vi "OscTest.vi"() -> ()   [LabVIEW 2017]
uses:
  <vilib>/Analysis/baseanly.llb/Mean (DBL).vi
  DS1054z.lvlib
  <vilib>/Analysis/NI_AALBase.lvlib
panel:
  out "Waveform Chart":u32(graph)
  out "Array":string[](array[string])
  out "OutData":cluster{string, "userdata":string}
  out "Waveform Graph 5":dbl[](graph)
  out "Waveform Graph 4":u32[](graph)
  out "mean":dbl format="%0.2f"
  out "Waveform Graph 3":dbl[](graph)
  out "Numeric":i32
  out "x-y":u32
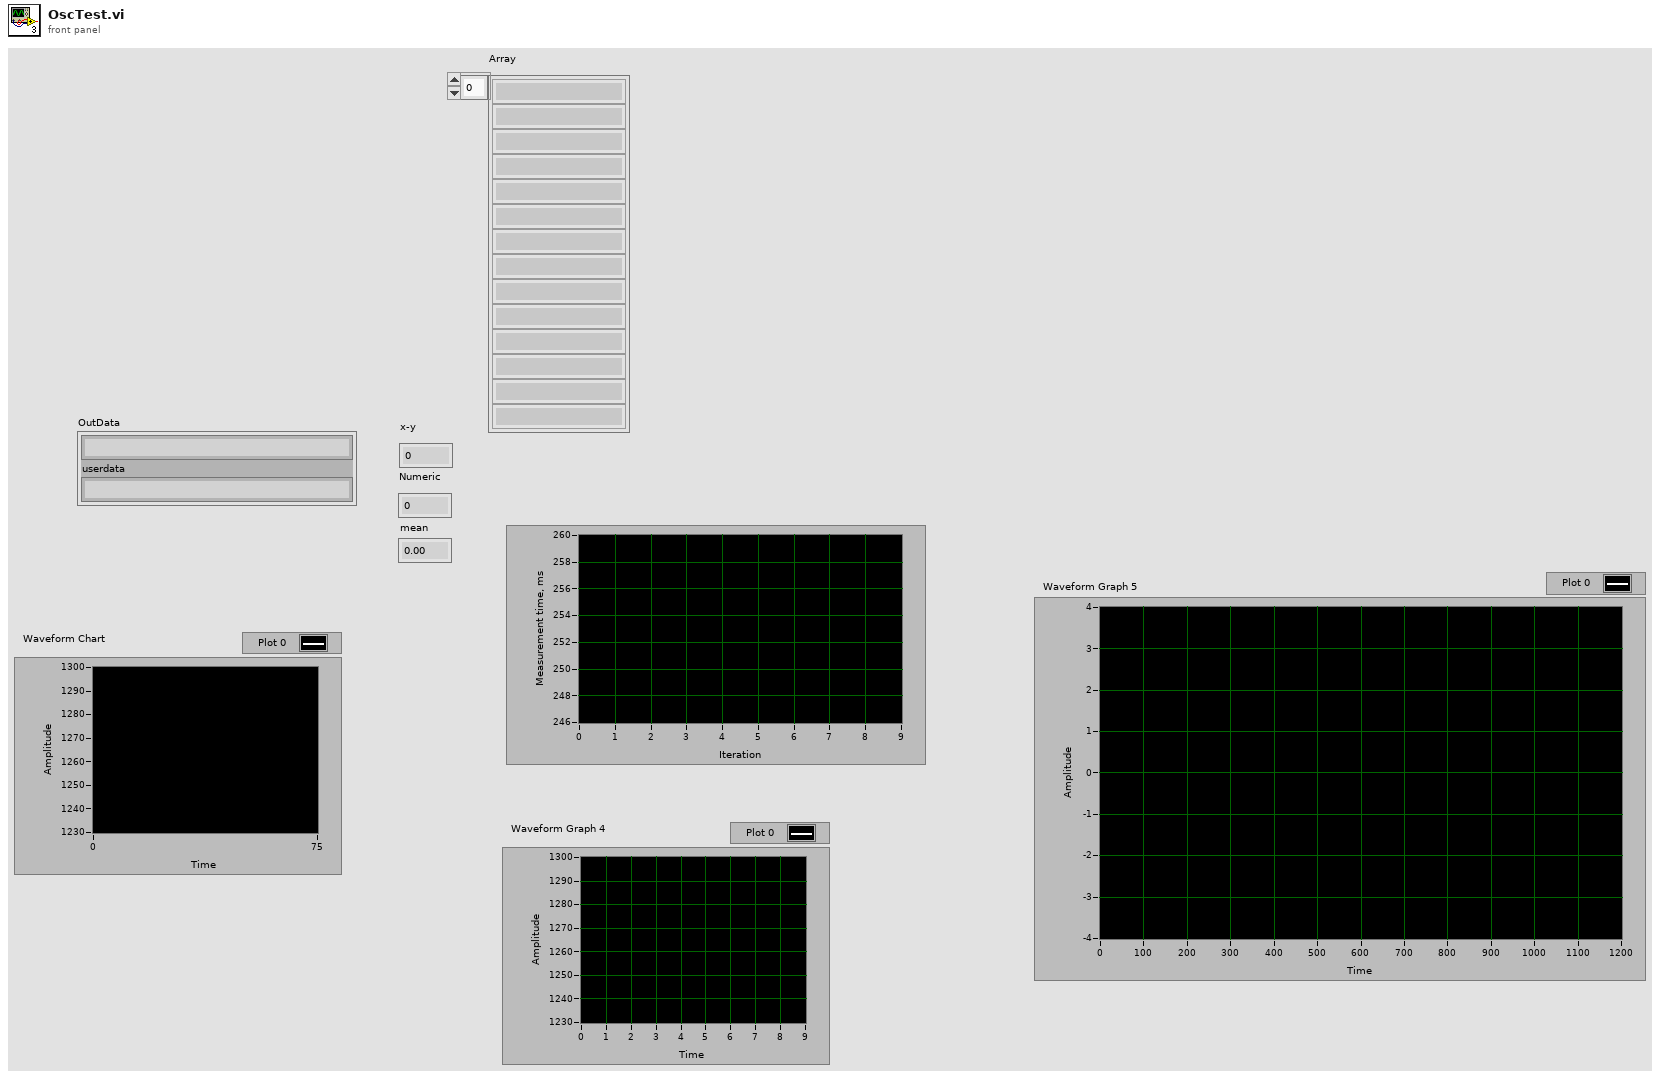
[diagram p1: front panel]
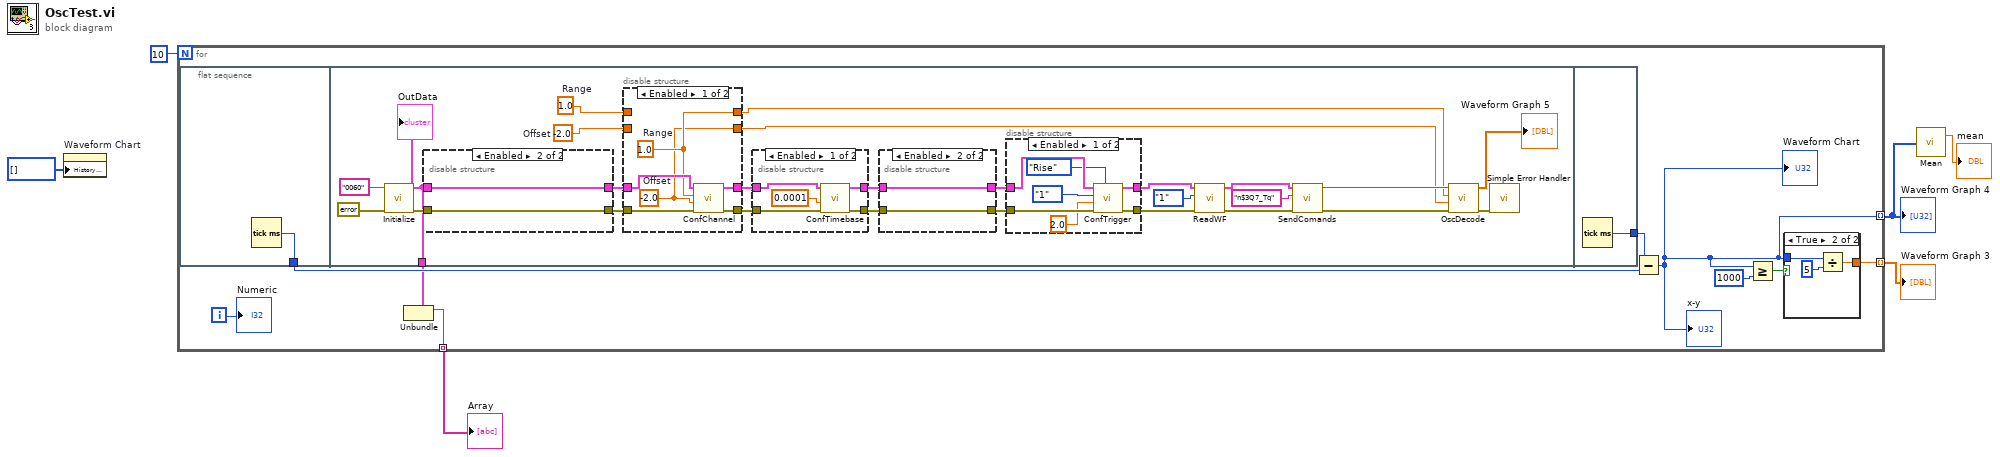
[diagram p0: block diagram]
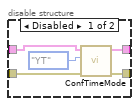
[diagram p4: hidden frame]
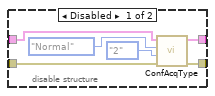
[diagram p7: hidden frame]
diagram:
  n1 = property on="Waveform Chart" class="WFChart (strict)"("History Data"=u32[] []) -> ()  [unwired: 2 in, 2 out]
  n2 = for {
    N: 10 -> [_]
    tunnel: [w7] -> w1 mode=indexing
    tunnel: [w11] -> w4 mode=indexing
    tunnel: [w9] -> w3 mode=indexing
    i -> [w14]
    n3 = flat-sequence {
      tunnel: [w20] -> w15
      tunnel: [w21] -> w10
      tunnel: [w88] -> w8
      frame #0 {
        n4 = Tick Count (ms)() -> (millisecond timer value=w20:u32)
      }
      frame #1 {
        w22 = -2.0  # Offset
        w23 = 1.0  # Range
        n5 = call "Initialize.vi"("error in (no error)"=errorcluster {"status"=FALSE, "code"=0, "source"=""}, "UserID"="0060") -> ("error out"=w44:errorcluster, "OutData"=w21:cluster{string, "userdata":string})  [unwired: 8 in]
        "OutData" <- w21
        n6 = disable-structure shown="Enabled" {
          disable-tunnel: w21 -> [w85 w87]
          disable-tunnel: w44 -> [w84 w86]
          disable-tunnel: [w81 w87] -> w37
          disable-tunnel: [w80 w86] -> w36
          frame Disabled {
            n7 = call "ConfAcqType.vi"("error in"=w84, "NumOfAver"=enum16{"2", "4", "8", "16"}."2", "Type"=enum16{"Normal", "Average", "Peak Detect"}."Normal", "InputData"=w85) -> ("error out"=w80:errorcluster, "OutputData"=w81:cluster{"String":string, string})  [unwired: 6 in]
          }
          frame Enabled {
          }
        }
        n8 = disable-structure shown="Enabled" {
          disable-tunnel: w37 -> [w75 w79]
          disable-tunnel: w36 -> [w74 w78]
          disable-tunnel: [w73 w79] -> w35
          disable-tunnel: [w72 w78] -> w34
          disable-tunnel: [w71 w77] -> w25
          disable-tunnel: [w70 w76] -> w24
          disable-tunnel: w23 -> [_ w77]
          disable-tunnel: w22 -> [_ w76]
          frame Enabled {
            w70 = -2.0  # Offset
            w71 = 1.0  # Range
            n9 = call "ConfChannel.vi"("error in"=w74, "Offset"=w70, "Range"=w71, "InputData"=w75) -> ("error out"=w72:errorcluster, "OutputData"=w73:cluster{"String":string, string})  [unwired: 6 in]
          }
          frame Disabled {
          }
        }
        n10 = disable-structure shown="Enabled" {
          disable-tunnel: w35 -> [w67 w69]
          disable-tunnel: w34 -> [w66 w68]
          disable-tunnel: [w65 w69] -> w33
          disable-tunnel: [w64 w68] -> w32
          frame Enabled {
            n11 = call "ConfTimebase.vi"("error in"=w66, "Timebase"=0.0001, "InputData"=w67) -> ("error out"=w64:errorcluster, "OutputData"=w65:cluster{"String":string, string})  [unwired: 7 in]
          }
          frame Disabled {
          }
        }
        n12 = disable-structure shown="Enabled" {
          disable-tunnel: w33 -> [w60 w62]
          disable-tunnel: w32 -> [w59 w61]
          disable-tunnel: [w58 w62] -> w31
          disable-tunnel: [w57 w61] -> w30
          frame Disabled {
            n13 = call "ConfTimeMode.vi"("error in"=w59, "Timebase Mode"=enum16{"YT", "XY"}."YT", "InputData"=w60) -> ("error out"=w57:errorcluster, "OutputData"=w58:cluster{"String":string, string})  [unwired: 7 in]
          }
          frame Enabled {
          }
        }
        n14 = disable-structure shown="Enabled" {
          disable-tunnel: [w53 w55] -> w42
          disable-tunnel: [w52 w54] -> w40
          disable-tunnel: w31 -> [w51 w55]
          disable-tunnel: w30 -> [w50 w54]
          frame Enabled {
            n15 = call "ConfTrigger.vi"("Slope"=enum16{"Rise", "Fall", "Both"}."Rise", "error in"=w50, "Level"=2.0, "Source"=enum16{"1", "2", "3", "4"}."1", "InputData"=w51) -> ("error out"=w52:errorcluster, "OutputData"=w53:cluster{"String":string, string})  [unwired: 5 in]
          }
          frame Disabled {
          }
        }
        n16 = call "ReadWF.vi"("error in"=w40, "Source"=enum16{"1", "2", "3", "4"}."1", "InputData"=w42) -> ("error out"=w39:errorcluster, "OutputData"=w41:cluster{"String":string, string})  [unwired: 7 in]
        n17 = call "SendComands.vi"("error in (no error)"=w39, "Password"="n$3Q7_Tq", "InputData"=w41) -> ("error out"=w28:errorcluster, "Result"=w29:string)  [unwired: 6 in, 1 out]
        n18 = call "OscDecode.vi"("error in"=w28, "Offset"=w24, "Range"=w25, "ReceivedData"=w29) -> ("error out"=w27:errorcluster, "MeasuredData"=→"Waveform Graph 5":dbl[])  [unwired: 5 in, 1 out]
        n19 = call <vilib>:"Simple Error Handler.vi"("error in (no error)"=w27) -> ()  [unwired: 4 in, 5 out]
      }
      frame #2 {
        n20 = Tick Count (ms)() -> (millisecond timer value=w88:u32)
      }
    }
    n21 = Unbundle(w10) -> (w9:string)  [unwired: 1 out]
    n22 = Subtract(x=w8, y=w15) -> (x-y=w7:u32)
    "x-y" <- w7
    "Waveform Chart" <- w7
    n23 = Greater Or Equal?(x=w7, y=u32 1000) -> (x >= y?=w12:bool)
    n24 = case shown="True" w12 {
      tunnel: w7 -> [w16 w19]
      tunnel: [w16 w17] -> w11
      frame False {
      }
      frame True {
        n25 = Divide(x=w19, y=u32 5) -> (x/y=w17:dbl)
      }
    }
    "Numeric" <- w14
  }
  "Waveform Graph 3" <- w4
  "Waveform Graph 4" <- w1
  "Array" <- w3
  n26 = call-poly <vilib>:"Mean.vi"("X"=w1) -> ("mean"=→"mean":dbl)  [unwired: 1 out]
